vi "Grab Image.vi"(8 "error in":errorcluster, 11 "DMK33UP2000 in":refnum<class "DMK33UP2000.lvclass">) -> (0 "error out":errorcluster, 3 "DMK33UP2000 out":refnum<class "DMK33UP2000.lvclass">)   [LabVIEW 2018, in "DMK33UP2000.lvlib" / "DMK33UP2000.lvclass"]
uses:
  DMK33UP2000.lvclass
  builds/Camera.lvlibp/Camera.lvclass
  <vilib>/vision/driver/NI_Vision_Acquisition_Software.lvlib
  C:/Users/Ron.Dexter.LUMINARTECH/Desktop/builds/Camera.lvlibp/Camera.lvclass
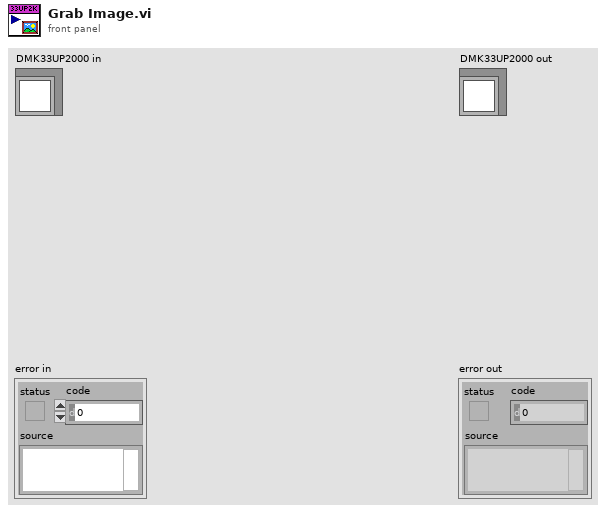
[diagram p1: front panel]
types:
  T1 = typedef "Camera.lvlibp/IMAQ Image.ctl" = refnum<image>
  T2 = typedef "Image Type" = u32
  T3 = typedef "IMAQ Image.ctl" = refnum<image>
  T4 = typedef "Camera.lvlibp/IMAQdx.ctl" = refnum<k21>
  T5 = typedef "IMAQdx.ctl" = refnum<k21>
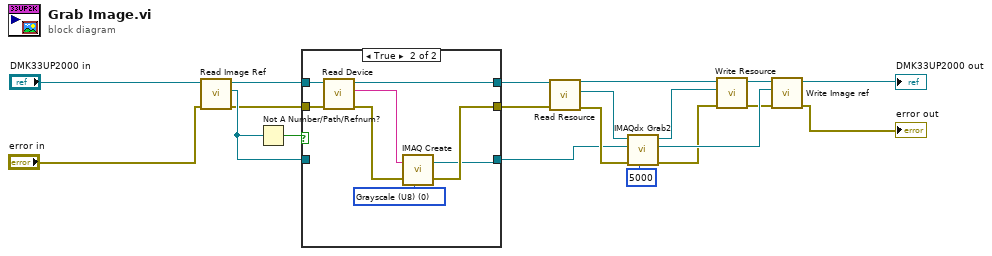
[diagram p0: block diagram]
diagram:
  n1 = call "Read Image Ref.vi"("error in (no error)"="error in", "Camera in"="DMK33UP2000 in") -> ("error out"=w3:errorcluster, "Image"=w6:T1, "Camera out"=w4:refnum<class "DMK33UP2000.lvclass">)  [unwired: 7 in]
  n2 = Not A Number/Path/Refnum?(number/path/refnum=w6) -> (NaN/Path/Refnum?=w7:bool)
  n3 = case shown="True" w7 {
    tunnel: w6 -> [w23 _]
    tunnel: [w23 w25] -> w5
    tunnel: w4 -> [w22 w31]
    tunnel: w3 -> [w21 w30]
    tunnel: [w22 w29] -> w2
    tunnel: [w21 w27] -> w1
    frame False {
    }
    frame True {
      w24 = T2 0 items=["Grayscale (U8)", "Grayscale (I16)", "Grayscale (SGL)", "Complex (CSG)", "RGB (U32)", "HSL (U32)", "RGB (U64)", "Grayscale (U16)"] ("Image Type")
      n4 = call "Read Device.vi"("error in (no error)"=w30, "Camera in"=w31) -> ("error out"=w28:errorcluster, "Device"=w26:string, "Camera out"=w29:refnum<class "DMK33UP2000.lvclass">)  [unwired: 7 in]
      n5 = call "IMAQ Create"("Image Name"=w26, "Image Type"=w24, "error in (no error)"=w28) -> ("New Image"=w25:T3, "error out"=w27:errorcluster)  [unwired: 2 in]
    }
  }
  n6 = call "Read Resource.vi"("error in (no error)"=w1, "Camera in"=w2) -> ("error out"=w9:errorcluster, "IMAQdx Session"=w19:T4, "Camera out"=w16:refnum<class "DMK33UP2000.lvclass">)  [unwired: 7 in]
  n7 = call <vilib>:"IMAQdx Grab2.vi"("Timeout (ms)"=5000, "error in"=w9, "Image In"=w5, "Session In"=w19) -> ("error out"=w8:errorcluster, "Image Out"=w14:T3, "Session Out"=w15:T5)  [unwired: 4 in, 1 out]
  n8 = call "Write Resource.vi"("error in (no error)"=w8, "IMAQdx Session"=w15, "Camera in"=w16) -> ("error out"=w13:errorcluster, "Camera out"=w12:refnum<class "DMK33UP2000.lvclass">)  [unwired: 7 in]
  n9 = call "Write Image ref.vi"("error in (no error)"=w13, "Image"=w14, "Camera in"=w12) -> ("error out"=→"error out":errorcluster, "Camera out"=→"DMK33UP2000 out":refnum<class "DMK33UP2000.lvclass">)  [unwired: 7 in]
